vi "Byte189_190 (SubVI).vi"(3 "Input String":string) -> (0 "OUTPUTS":T1, 1 "INPUTS":T2)   [LabVIEW 2024]
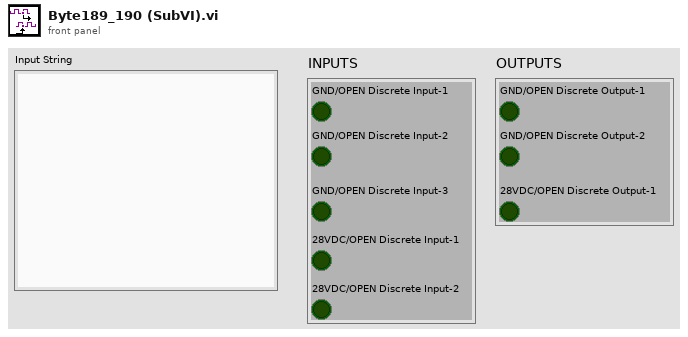
[diagram p1: front panel]
types:
  T1 = cluster{"GND/OPEN Discrete Output-1 ":bool, "GND/OPEN Discrete Output-2":bool, "28VDC/OPEN Discrete Output-1":bool}
  T2 = cluster{"GND/OPEN Discrete Input-1":bool, "GND/OPEN Discrete Input-2":bool, "GND/OPEN Discrete Input-3":bool, "28VDC/OPEN Discrete Input-1":bool, "28VDC/OPEN Discrete Input-2":bool}
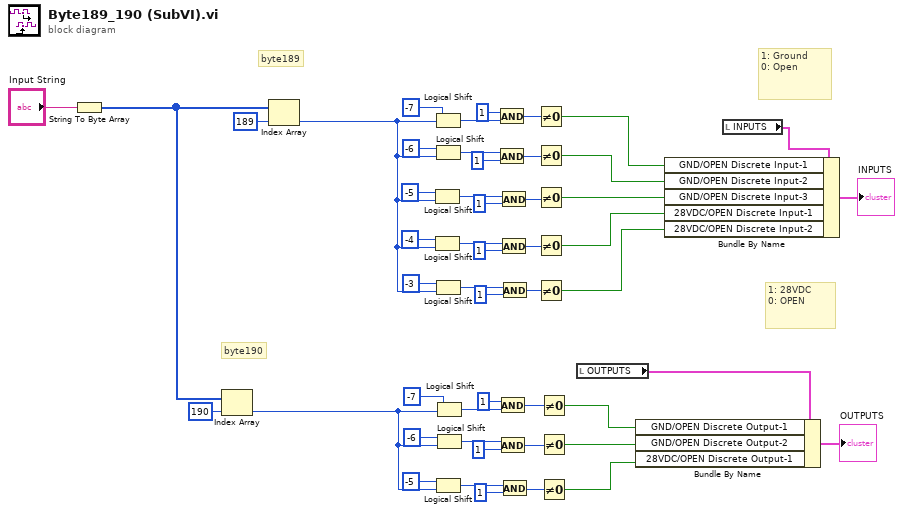
[diagram p0: block diagram]
diagram:
  # "byte190"
  # "1: Ground\n0: Open"
  # "1: 28VDC\n0: OPEN"
  # "byte189"
  n1 = String To Byte Array(string="Input String") -> (unsigned byte array=w31:u8[])
  n2 = Index Array "Index Array"(array=w31, index=190) -> (element=w21:u8)
  n3 = Index Array "Index Array"(array=w31, index=189) -> (element=w33:u8)
  n4 = Logical Shift(y=i16 -5, x=w33) -> (x << y=w45:u8)
  n5 = Logical Shift(y=i16 -4, x=w33) -> (x << y=w37:u8)
  n6 = Logical Shift(y=i16 -7, x=w33) -> (x << y=w41:u8)
  n7 = Logical Shift(y=i16 -6, x=w33) -> (x << y=w43:u8)
  n8 = Logical Shift(y=i16 -3, x=w33) -> (x << y=w34:u8)
  n9 = Logical Shift(y=i16 -5, x=w21) -> (x << y=w27:u8)
  n10 = Logical Shift(y=i16 -7, x=w21) -> (x << y=w23:u8)
  n11 = Logical Shift(y=i16 -6, x=w21) -> (x << y=w25:u8)
  n12 = And(x=u16 1, y=w41) -> (x .and. y?=w20:u16)
  n13 = And(x=w43, y=u16 1) -> (x .and. y?=w19:u16)
  n14 = And(x=u16 1, y=w23) -> (x .and. y?=w15:u16)
  n15 = And(x=w25, y=u16 1) -> (x .and. y?=w14:u16)
  n16 = And(x=w45, y=u16 1) -> (x .and. y?=w18:u16)
  n17 = And(x=w37, y=u16 1) -> (x .and. y?=w17:u16)
  n18 = And(x=w34, y=u16 1) -> (x .and. y?=w16:u16)
  n19 = And(x=w27, y=u16 1) -> (x .and. y?=w13:u16)
  n20 = Not Equal To 0?(x=w20) -> (x != 0?=w10:bool)
  n21 = Not Equal To 0?(x=w19) -> (x != 0?=w11:bool)
  n22 = Not Equal To 0?(x=w18) -> (x != 0?=w12:bool)
  n23 = Not Equal To 0?(x=w17) -> (x != 0?=w9:bool)
  n24 = Not Equal To 0?(x=w16) -> (x != 0?=w8:bool)
  n25 = Not Equal To 0?(x=w15) -> (x != 0?=w4:bool)
  n26 = Not Equal To 0?(x=w14) -> (x != 0?=w5:bool)
  n27 = Not Equal To 0?(x=w13) -> (x != 0?=w3:bool)
  n28 = local read "OUTPUTS"() -> (w2:T1)
  n29 = Bundle By Name(cluster=w2, "GND/OPEN Discrete Output-1"=w4, "GND/OPEN Discrete Output-2"=w5, "28VDC/OPEN Discrete Output-1"=w3) -> (→"OUTPUTS":T1)
  n30 = local read "INPUTS"() -> (w7:T2)
  n31 = Bundle By Name(cluster=w7, "GND/OPEN Discrete Input-1"=w10, "GND/OPEN Discrete Input-2"=w11, "GND/OPEN Discrete Input-3"=w12, "28VDC/OPEN Discrete Input-1"=w9, "28VDC/OPEN Discrete Input-2"=w8) -> (→"INPUTS":T2)
